vi "Create Result Name.vi"(9 "AlgSet":string, 11 "ROIList":string[](array[string])) -> (3 "AlgResultName":string[](array[string]))   [LabVIEW 2019]
uses:
  Analysis/Controls/Analysis_Setting.ctl
  Analysis/Controls/V_Analysis_Type.ctl
  Analysis/Controls/Color Pattern Match/Analysis Color Pattern Match Parameter.ctl
  Analysis/Controls/Parttern Match/Analysis_PatternMatch_Parameter.ctl
  Analysis/Controls/Geometric Match/Analysis_Geometric PatternMatch_Parameter.ctl
  <vilib>/vision/Pattern Matching.llb/IMAQ Match Range Setting.ctl
  Analysis/Controls/ShapeDectect/Analysis_ShapeDectect_Parameter.ctl
  06c4f6b3-c99a-474d-8418-8735cb839037.vi
  58aaab81-13dd-4ef9-b524-eb528f82a9b5.vi
  56b1ed83-df22-40c3-9242-75fec88c9c5b.vi
  9e2b9a15-3d4d-495b-819c-c3aed1fd0666.vi
  aeadb3aa-3f99-46f6-b047-b8eaad8a81a3.vi
  <vilib>/JDP Science/JSONtext/JSON text to Variant.vi
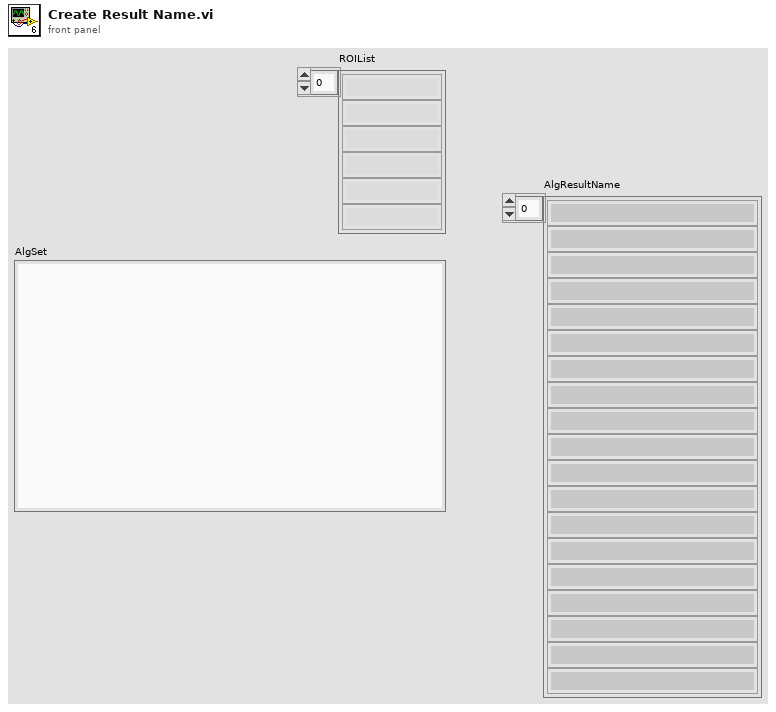
[diagram p1: front panel]
types:
  T1 = typedef "Analysis_Setting.ctl" = cluster{"PreProcess":T2, "Parameter":string}
  T2 = typedef "V_Analysis_Type.ctl" = enum16{"None", "C_Color Pattern Matching", "G_PatternMatching", "G_ShapeDectect", "G_GeometricMatch", "B_Area Check"}
  T3 = typedef "Analysis Color Pattern Match Parameter.ctl" = cluster{"IgnoreBlack And White":enum16{"Disable", "IgnoreBlack", "IgnoreWhite", "IgnoreBlack And White"}, "Match Saturation Threshold":i32, "Minimum Match Score":i32, "Color Score Weight":i32, "Color Sensitivity":u32, "Search Strategy":u32, "Match Offset":cluster{"X":dbl, "Y":dbl}, "Number of Matches to Find":i32, "AngleRange+/-":dbl, "Sub-Pixel Accuracy":bool, "ROI Descriptor":T4, "TemplatePath":string, "Match Mode":enum16{"Shift Invariant", "Rotation Invariant"}}
  T4 = typedef "ROI Descriptor" = cluster{"Global Rectangle":i32[], "Contours":cluster{"ID":enum32{"External", "Internal"}, "Type":u32, "Coordinates":i32[]}[]}
  T5 = typedef "Analysis_PatternMatch_Parameter.ctl" = cluster{"Algorithm":i32, "Match Parameters":cluster{"Number of Matches Requested":i32, "Minimum Match Score":sgl, "Angle Ranges":cluster{"Start Angle":sgl, "End Angle":sgl}[]}, "ROI Descriptor":T4, "Advanced Options":cluster{"Item":u16, "Value":dbl}[], "Template path":string, "XOffset":i32, "YOffset":i32}
  T6 = typedef "Analysis_Geometric PatternMatch_Parameter.ctl" = cluster{"Curve Extraction":cluster{"Extraction Mode":u32, "Edge Threshold":i32, "Edge Filter Size":u32, "Min Length":i32, "Row Search Step Size":i32, "Column Search Step Size":i32, "Max Endpoint Gap":i32, "Closed":bool, "Subpixel":bool}, "X Position Offset":i32, "Y Position Offset":i32, "Match Parameters":cluster{"Number of Matches Requested":i32, "Minimum Match Score":sgl, "Angle Ranges":cluster{"Start Angle":sgl, "End Angle":sgl}[]}, "Template path":string, "Range Settings":T7[], "Match Mode":cluster{"Rotation":bool, "Scale":bool, "Occlusion":bool, "Reserved":bool, "Reserved":bool, "Reserved":bool}}
  T7 = typedef "IMAQ Match Range Setting.ctl" = cluster{"Match Constraints":u32, "Min":dbl, "Max":dbl}
  T8 = typedef "Analysis_ShapeDectect_Parameter.ctl" = cluster{"Enum_ShapeType":enum16{"Circles", "Ellipses", "Lines", "Rectangles"}, "MaxParticle":i32, "Descriptor":cluster{"Set 1":dbl, "Set 2":dbl, "Set 3":dbl, "Set 4":dbl}, "Match Options":cluster{"Rotation":bool, "Scale":bool, "Occlusion":bool, "Range Settings":cluster{"Match Constraints":u32, "Min":dbl, "Max":dbl}[]}, "Curve Parameters":cluster{"Extraction Mode":u32, "Edge Threshold":i32, "Edge Filter Size":u32, "Min Length":i32, "Row Search Step Size":i32, "Col Search Step Size":i32, "Max Endpoint Gap":i32, "Closed":bool, "Subpixel":bool}, " score":dbl}
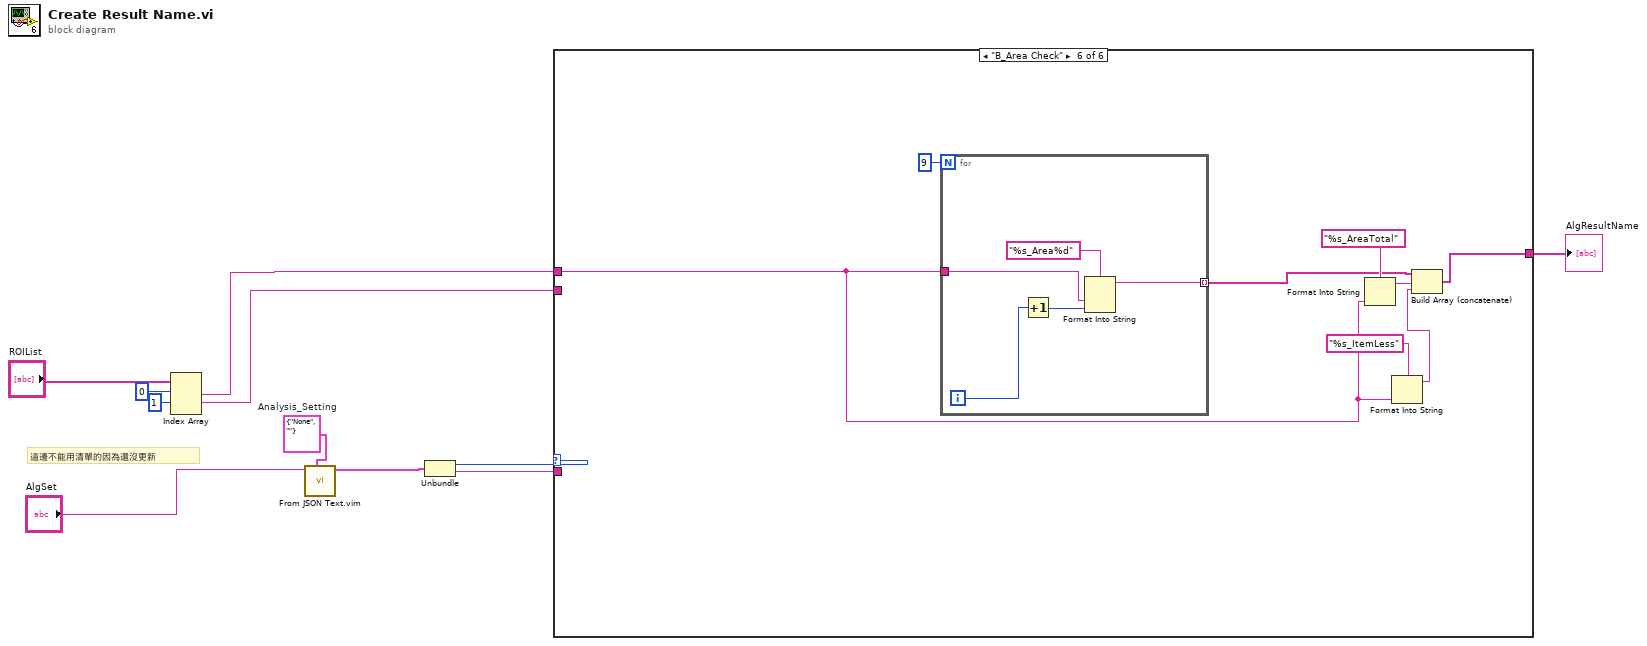
[diagram p0: block diagram]
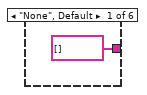
[diagram p2: hidden frame]
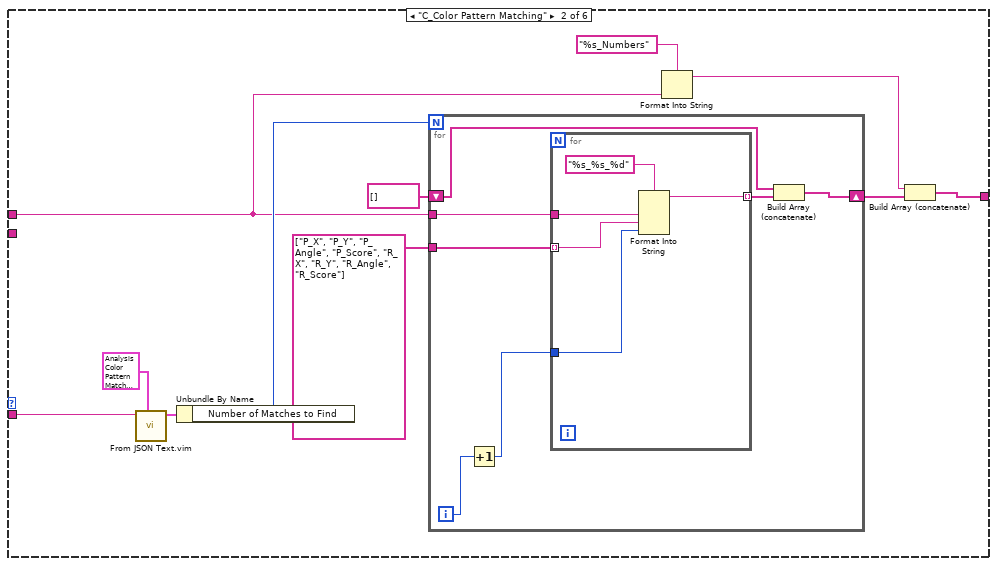
[diagram p3: hidden frame]
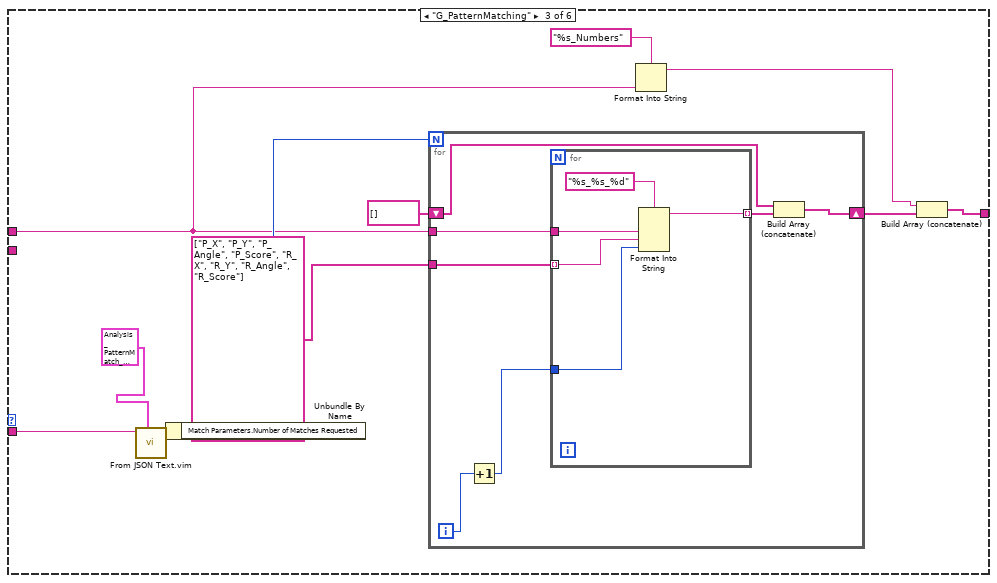
[diagram p4: hidden frame]
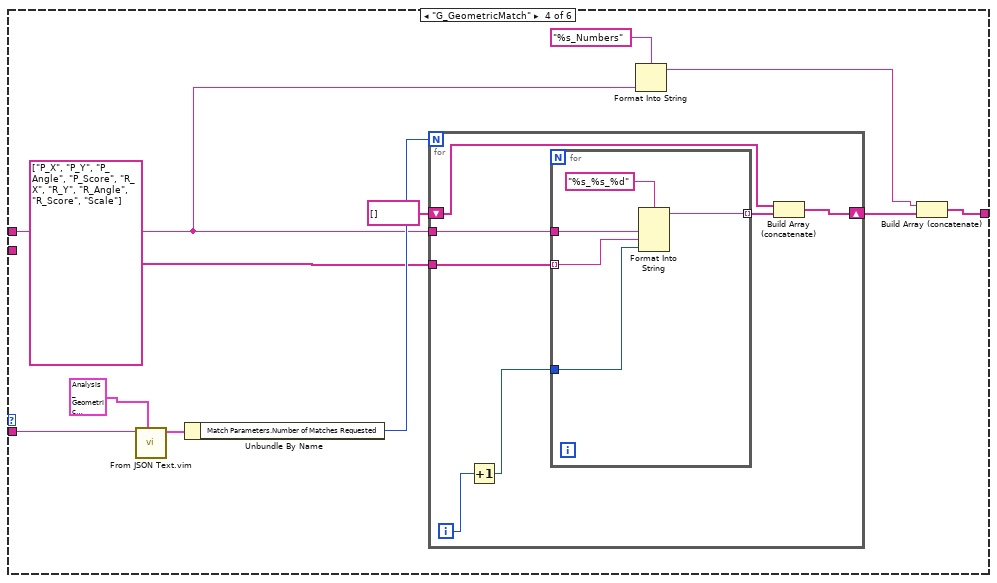
[diagram p5: hidden frame]
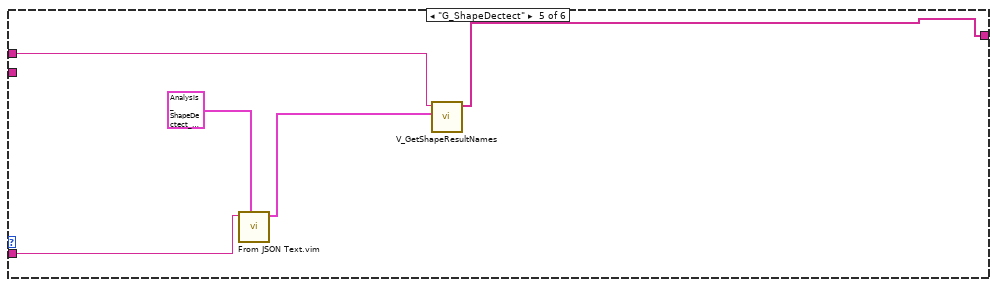
[diagram p6: hidden frame]
diagram:
  w9 = T1 {"PreProcess"=enum."None", "Parameter"=""}  # Analysis_Setting
  # "這邊不能用清單的因為還沒更新"
  n1 = Index Array(array="ROIList", index #1=0 ("index"), index #2=1 ("index")) -> (element #1=w6:string, element #2=w4:string)  [unwired: 1 in, 1 out]
  n2 = call "From JSON Text.vim"("Data Type and Default Value"=w9, "JSON"="AlgSet") -> ("Data out"=w7:T1)  [unwired: 8 in, 1 out]
  n3 = Unbundle(w7) -> ("PreProcess"=w2:T2, "Parameter"=w8:string)
  n4 = case shown="\"B_Area Check\"" w2 {
    tunnel: w8 -> [_ w23 w46 w69 w85 _]
    tunnel: w6 -> [_ w15 w41 w64 w84 w87]
    tunnel: w4 -> [_ _ _ _ _ _]
    tunnel: [string[] [] w14 w40 w63 w83 w90] -> w3
    frame "None", Default {
    }
    frame "C_Color Pattern Matching" {
      n5 = call "From JSON Text.vim"("Data Type and Default Value"=T3 {"IgnoreBlack And White"=enum."IgnoreBlack And White", "Match Saturation Threshold"=80, "Minimum Match Score"=750, "Color Score Weight"=750, "Color Sensitivity"=1, "Search Strategy"=0, "Match Offset"={"X"=0.0, "Y"=0.0}, "Number of Matches to Find"=0, "AngleRange+/-"=0.0, "Sub-Pixel Accuracy"=FALSE, "ROI Descriptor"={"Global Rectangle"=[], "Contours"=[]}, "TemplatePath"="", "Match Mode"=enum."Rotation Invariant"} ("Color Pattern Match"), "JSON"=w23) -> ("Data out"=w21:T3)  [unwired: 8 in, 1 out]
      n6 = Unbundle By Name(w21) -> ("Number of Matches to Find"=w18:i32)
      n7 = for {
        N: w18 -> [_]
        tunnel: w15 -> [w30]
        tunnel: string[] ["P_X", "P_Y", "P_Angle", "P_Score", "R_X", "R_Y", "R_Angle", "R_Score"] -> [w29]
        shift-right: [w25] -> w17
        shift-left: string[] [] -> [w24]
        i -> [w28]
        n8 = Increment(x=w28) -> (x+1=w27:i32)
        n9 = for {
          tunnel: w30 -> [w34]
          tunnel: w29 -> [w33] mode=indexing
          tunnel: w27 -> [w32]
          tunnel: [w31] -> w26 mode=indexing
          n10 = Format Into String(format string="%s_%s_%d", w34, w33, w32) -> (resulting string=w31:string)  [unwired: 2 in, 1 out]
        }
        n11 = Build Array (concatenate)(w24, w26) -> (w25:string[])
      }
      n12 = Format Into String(format string="%s_Numbers", w15) -> (resulting string=w13:string)  [unwired: 2 in, 1 out]
      n13 = Build Array (concatenate)(w13, w17) -> (w14:string[])
    }
    frame "G_PatternMatching" {
      n14 = call "From JSON Text.vim"("Data Type and Default Value"=T5 {"Algorithm"=2, "Match Parameters"={"Number of Matches Requested"=1, "Minimum Match Score"=750.0, "Angle Ranges"=[]}, "ROI Descriptor"={"Global Rectangle"=[], "Contours"=[]}, "Advanced Options"=[{"Item"=1, "Value"=1.0}, {"Item"=103, "Value"=1.0}], "Template path"="", "XOffset"=0, "YOffset"=0} ("PatternMatchParameter"), "JSON"=w46) -> ("Data out"=w38:T5)  [unwired: 8 in, 1 out]
      n15 = Unbundle By Name(w38) -> ("Match Parameters.Number of Matches Requested"=w44:i32)
      n16 = for {
        N: w44 -> [_]
        tunnel: w41 -> [w53]
        tunnel: string[] ["P_X", "P_Y", "P_Angle", "P_Score", "R_X", "R_Y", "R_Angle", "R_Score"] -> [w52]
        shift-right: [w48] -> w43
        shift-left: string[] [] -> [w47]
        i -> [w51]
        n17 = Increment(x=w51) -> (x+1=w50:i32)
        n18 = for {
          tunnel: w53 -> [w57]
          tunnel: w52 -> [w56] mode=indexing
          tunnel: w50 -> [w55]
          tunnel: [w54] -> w49 mode=indexing
          n19 = Format Into String(format string="%s_%s_%d", w57, w56, w55) -> (resulting string=w54:string)  [unwired: 2 in, 1 out]
        }
        n20 = Build Array (concatenate)(w47, w49) -> (w48:string[])
      }
      n21 = Format Into String(format string="%s_Numbers", w41) -> (resulting string=w39:string)  [unwired: 2 in, 1 out]
      n22 = Build Array (concatenate)(w39, w43) -> (w40:string[])
    }
    frame "G_GeometricMatch" {
      n23 = call "From JSON Text.vim"("Data Type and Default Value"=T6 {"Curve Extraction"={"Extraction Mode"=0, "Edge Threshold"=75, "Edge Filter Size"=1, "Min Length"=25, "Row Search Step Size"=15, "Column Search Step Size"=15, "Max Endpoint Gap"=10, "Closed"=FALSE, "Subpixel"=FALSE}, "X Position Offset"=0, "Y Position Offset"=0, "Match Parameters"={"Number of Matches Requested"=1, "Minimum Match Score"=750.0, "Angle Ranges"=[]}, "Template path"="", "Range Settings"=[], "Match Mode"={"Rotation"=TRUE, "Scale"=FALSE, "Occlusion"=FALSE, "Reserved"=FALSE, "Reserved"=FALSE, "Reserved"=FALSE}} ("Cluster"), "JSON"=w69) -> ("Data out"=w61:T6)  [unwired: 8 in, 1 out]
      n24 = Unbundle By Name(w61) -> ("Match Parameters.Number of Matches Requested"=w67:i32)
      n25 = for {
        N: w67 -> [_]
        tunnel: w64 -> [w76]
        tunnel: string[] ["P_X", "P_Y", "P_Angle", "P_Score", "R_X", "R_Y", "R_Angle", "R_Score", "Scale"] -> [w75]
        shift-right: [w71] -> w66
        shift-left: string[] [] -> [w70]
        i -> [w74]
        n26 = Increment(x=w74) -> (x+1=w73:i32)
        n27 = for {
          tunnel: w76 -> [w80]
          tunnel: w75 -> [w79] mode=indexing
          tunnel: w73 -> [w78]
          tunnel: [w77] -> w72 mode=indexing
          n28 = Format Into String(format string="%s_%s_%d", w80, w79, w78) -> (resulting string=w77:string)  [unwired: 2 in, 1 out]
        }
        n29 = Build Array (concatenate)(w70, w72) -> (w71:string[])
      }
      n30 = Format Into String(format string="%s_Numbers", w64) -> (resulting string=w62:string)  [unwired: 2 in, 1 out]
      n31 = Build Array (concatenate)(w62, w66) -> (w63:string[])
    }
    frame "G_ShapeDectect" {
      n32 = call "From JSON Text.vim"("Data Type and Default Value"=T8 {"Enum_ShapeType"=enum."Circles", "MaxParticle"=1, "Descriptor"={"Set 1"=10.0, "Set 2"=100.0, "Set 3"=200.0, "Set 4"=10.0}, "Match Options"={"Rotation"=TRUE, "Scale"=FALSE, "Occlusion"=FALSE, "Range Settings"=[{"Match Constraints"=0, "Min"=0.0, "Max"=360.0}]}, "Curve Parameters"={"Extraction Mode"=0, "Edge Threshold"=75, "Edge Filter Size"=1, "Min Length"=25, "Row Search Step Size"=15, "Col Search Step Size"=15, "Max Endpoint Gap"=10, "Closed"=FALSE, "Subpixel"=FALSE}, " score"=500.0} ("ShapeDetectParameter"), "JSON"=w85) -> ("Data out"=w82:T8)  [unwired: 8 in, 1 out]
      n33 = call "V_GetShapeResultNames.vi"("SetParameter"=w82, "ROI_Name"=w84) -> ("ResultNames"=w83:string[])  [unwired: 9 in]
    }
    frame "B_Area Check" {
      n34 = for {
        N: 9 -> [_]
        tunnel: w87 -> [w98]
        tunnel: [w95] -> w91 mode=indexing
        i -> [w97]
        n35 = Increment(x=w97) -> (x+1=w96:i32)
        n36 = Format Into String(format string="%s_Area%d", w98, w96) -> (resulting string=w95:string)  [unwired: 2 in, 1 out]
      }
      n37 = Format Into String(format string="%s_AreaTotal", w87) -> (resulting string=w92:string)  [unwired: 2 in, 1 out]
      n38 = Format Into String(format string="%s_ItemLess", w87) -> (resulting string=w88:string)  [unwired: 2 in, 1 out]
      n39 = Build Array (concatenate)(w91, w92, w88) -> (w90:string[])
    }
  }
  "AlgResultName" <- w3
